vi "correlation_noise_gen.vi"(10 "噪声方差":dbl=0.5, 11 "观测时刻（0-1）":dbl[](array[numeric])) -> (3 "平均观测噪声":dbl format="%0.2f")   [LabVIEW 2018]
uses:
  <vilib>/Analysis/baseanly.llb/Mean (DBL).vi
  <vilib>/ptbypt/NI_PtbyPt.lvlib
  <vilib>/Analysis/NI_AALBase.lvlib
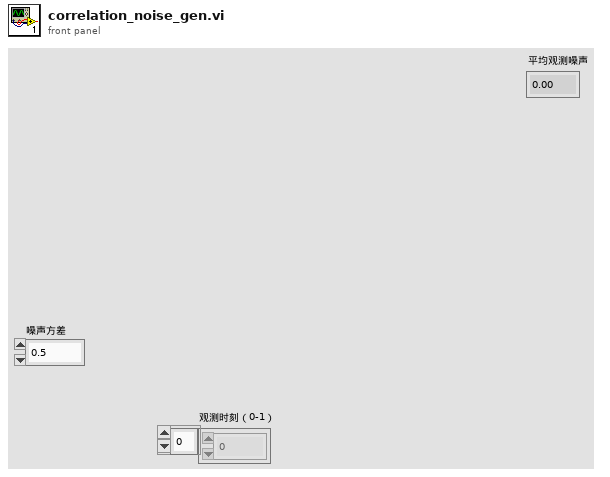
[diagram p1: front panel]
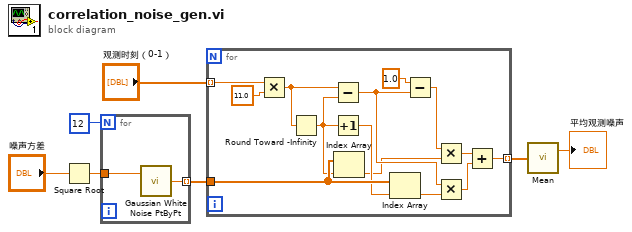
[diagram p0: block diagram]
diagram:
  n1 = Square Root(x="噪声方差") -> (sqrt(x)=w5:dbl)
  n2 = for {
    N: 12 -> [_]
    tunnel: w5 -> [w9]
    tunnel: [w8] -> w4 mode=indexing
    n3 = call <vilib>:"Gaussian White Noise PtByPt.vi"("standard deviation"=w9) -> ("Gaussian white noise"=w8:dbl)  [unwired: 2 in]
  }
  n4 = for {
    tunnel: "观测时刻（0-1）" -> [w23] mode=indexing
    tunnel: w4 -> [w20]
    tunnel: [w10] -> w2 mode=indexing
    n5 = Multiply(x=w23, y=11.0) -> (x*y=w21:dbl)
    n6 = Round Toward -Infinity(1:w21) -> (0:w19:dbl)
    n7 = Subtract(x=w21, y=w19) -> (x-y=w16:dbl)
    n8 = Increment(x=w19) -> (x+1=w18:dbl)
    n9 = Index Array(array=w20, index=w19) -> (element=w14:dbl)
    n10 = Index Array(array=w20, index=w18) -> (element=w17:dbl)
    n11 = Subtract(x=1.0, y=w16) -> (x-y=w13:dbl)
    n12 = Multiply(x=w13, y=w14) -> (x*y=w12:dbl)
    n13 = Multiply(x=w16, y=w17) -> (x*y=w11:dbl)
    n14 = Add(x=w12, y=w11) -> (x+y=w10:dbl)
  }
  n15 = call-poly <vilib>:"Mean.vi"("X"=w2) -> ("mean"=→"平均观测噪声":dbl)  [unwired: 1 out]
